vi "ArduinoMeasureWrite.vi"(0 "Arduino adress":refnum<visa-resource-name>="COM4", 4 "Measurement delay [s]":u32=5, 7 "error in":errorcluster) -> (17 "Average RH [%]":dbl, 19 "Average temperature [°C]":dbl, 21 "Temperature [°C]":dbl, 22 "Min temperature [°C]":dbl, 23 "Max temperature [°C]":dbl, 24 "Rel. Humidity [%]":dbl, 25 "Min RH [%]":dbl, 26 "Max RH [%]":dbl, 27 "error out":errorcluster)   [LabVIEW 2018]
doc: "Reads temperature and rel. humidity using arduino and creates a waveform graph with while loop iteration number on the x-axis, temperature on y1 axis and rel. humidity on the y2 axis."
panel:
  out "time":string
  out "output file refnum":refnum<file>
  in  "Select folder to save data":path=path "C:/Users/itkstriplabview3/Documents/TRH"
  in  "stop":bool
  out "Start time":timestamp
  out "Temp. & RH":cluster{dbl[], dbl[]}[](graph)
  out "Last 10 measurements":string[][](table)
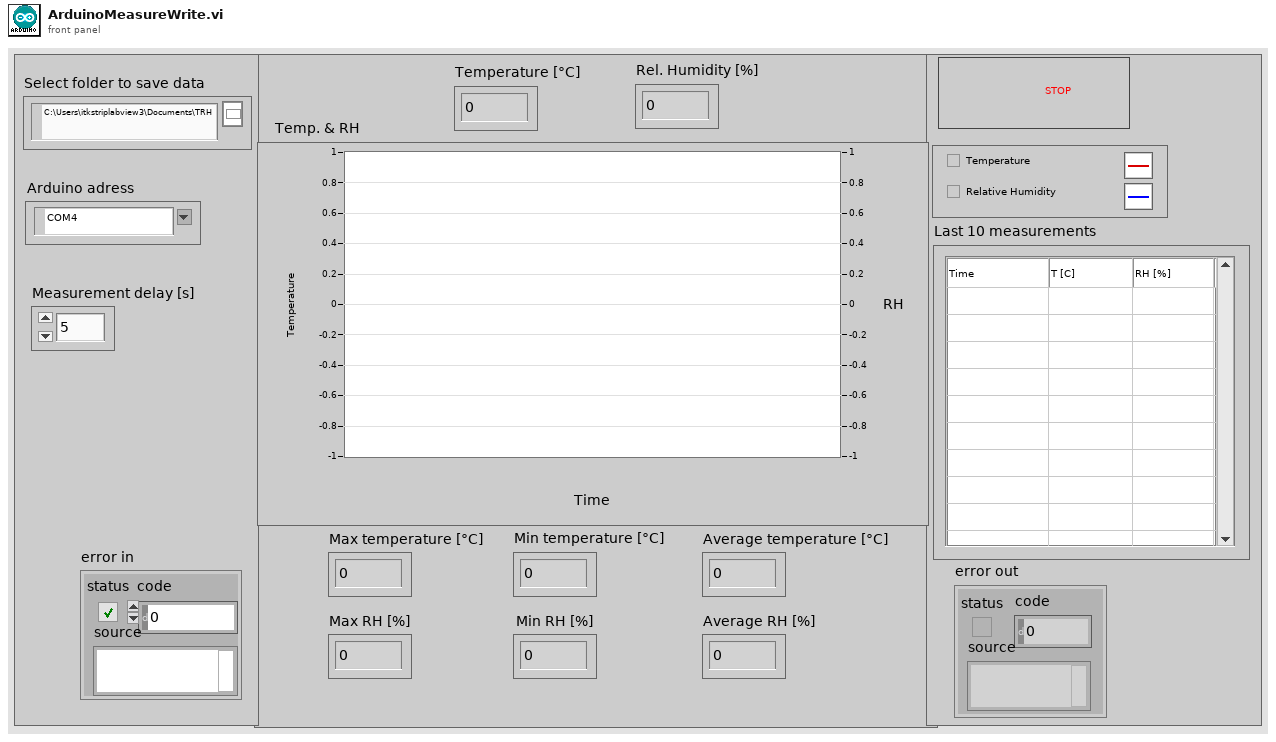
[diagram p1: front panel]
types:
  T1 = enum16{"open", "replace", "create", "open or create", "replace or create", "replace or create with confirmation"}
  T2 = typedef "LVDateTimeRec.ctl" = cluster{"fractional second":dbl, "second":i32, "minute":i32, "hour":i32, "day of month":i32, "month":i32, "year":i32, "day of week":i32, "day of year":i32, "DST":i32}
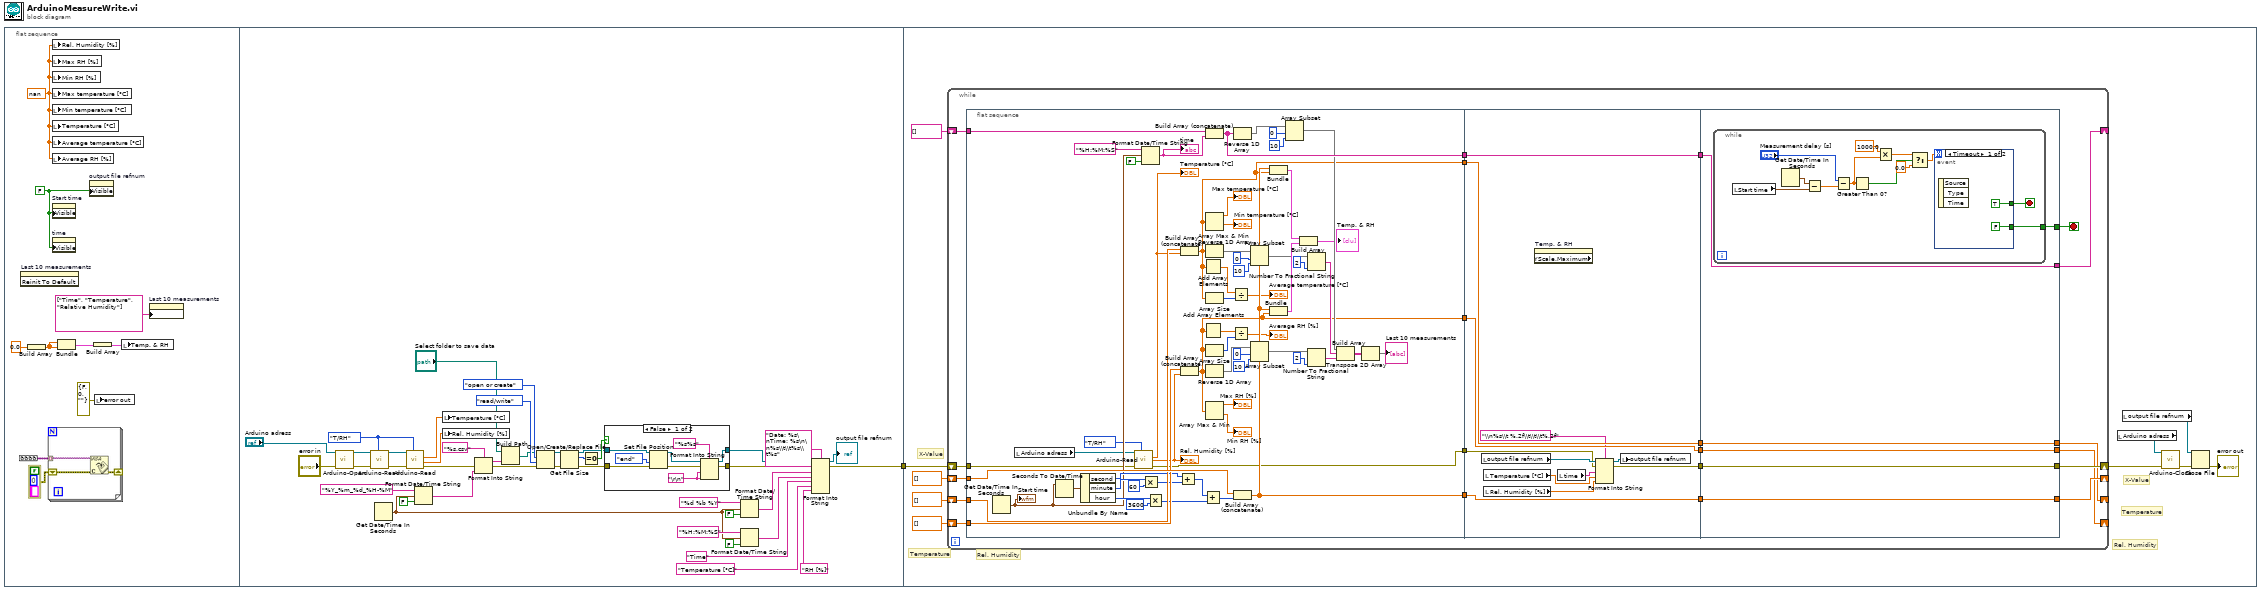
[diagram p0: block diagram]
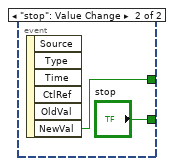
[diagram p3: hidden frame]
diagram:
  n1 = flat-sequence {
    tunnel: [w15] -> w1
    tunnel: w1 -> [w66]
    frame #0 {
      w3 = FALSE ("Visible")
      w6 = nan
      n2 = invoke on="Last 10 measurements" class="Tbl (strict)" method="Reinit To Default"() -> ()  [unwired: 3 in, 3 out]
      n3 = Build Array(0.0) -> (w8:dbl[])
      n4 = local write "Rel. Humidity [%]"(w6) -> ()
      n5 = local write "Max RH [%]"(w6) -> ()
      n6 = local write "Min RH [%]"(w6) -> ()
      n7 = local write "Max temperature [°C]"(w6) -> ()
      n8 = local write "Min temperature [°C]"(w6) -> ()
      n9 = local write "Temperature [°C]"(w6) -> ()
      n10 = local write "Average temperature [°C]"(w6) -> ()
      n11 = local write "Average RH [%]"(w6) -> ()
      n12 = property on="Start time" class="AbsTime (strict)"("Visible"=w3) -> ()  [unwired: 2 in, 2 out]
      n13 = property on="time" class="Str"("Visible"=w3) -> ()  [unwired: 2 in, 2 out]
      n14 = Bundle(w8, w8) -> (w7:cluster{dbl[], dbl[]})  [unwired: 1 in]
      n15 = property on="output file refnum" class="Ref (strict)"("Visible"=w3) -> ()  [unwired: 2 in, 2 out]
      n16 = Build Array(w7) -> (w9:cluster{dbl[], dbl[]}[])
      n17 = local write "error out"(errorcluster {"status"=FALSE, "code"=0, "source"=""} ("error out")) -> ()
      n18 = local write "Temp. & RH"(w9) -> ()
      n19 = property on="Last 10 measurements" class="Tbl (strict)"("Column Headers[]"=string[] ["Time", "Temperature", "Relative Humidity"]) -> ()  [unwired: 2 in, 2 out]
    }
    frame #1 {
      w42 = enum16{"T/RH", "Interlock", "Edgesense"}."T/RH" ("Arduino function")
      n20 = call "Arduino-Open.vi"("error in (no error)"="error in", "Visa Resource"="Arduino adress") -> ("error out"=w45:errorcluster, "VISA resource name out"=w47:refnum<visa-resource-name>)  [unwired: 7 in, 1 out]
      n21 = call "Arduino-Read.vi"("Arduino function"=w42, "error in (no error)"=w45, "VISA resource name"=w47) -> ("error out"=w46:errorcluster, "VISA resource name out"=w48:refnum<visa-resource-name>)  [unwired: 3 in, 4 out]
      n22 = Get Date/Time In Seconds() -> (seconds since 1Jan1904=w17:timestamp)
      n23 = call "Arduino-Read.vi"("Arduino function"=w42, "error in (no error)"=w46, "VISA resource name"=w48) -> ("error out"=w10:errorcluster, "rel. Humidity [%]"=w49:dbl, "Temperature [°C]"=w50:dbl)  [unwired: 3 in, 3 out]
      n24 = Format Date/Time String(time format string (%c)="%Y_%m_%d_%H-%M", seconds (now)=w17, UTC format=FALSE) -> (date/time string=w24:string)
      n25 = local write "Temperature [°C]"(w50) -> ()
      n26 = local write "Rel. Humidity [%]"(w49) -> ()
      n27 = Format Into String(format string="%s.csv", error in=w10, w24) -> (resulting string=w38:string, error out=w37:errorcluster)  [unwired: 1 in]
      n28 = Build Path(base path="Select folder to save data", name or relative path=w38) -> (appended path=w36:path)
      n29 = Open/Create/Replace File(file path (use dialog)=w36, error in=w37, operation (0:open)=T1."open or create", access (0:read/write)=enum16{"read/write", "read-only", "write-only"}."read/write") -> (refnum out=w34:refnum<file>, error out=w33:errorcluster)  [unwired: 2 in, 1 out]
      n30 = Get File Size(file=w34, error in=w33) -> (refnum out=w30:refnum<file>, size (in bytes)=w32:i64, 0:w29:errorcluster)
      n31 = Equal To 0?(x=w32) -> (x = 0?=w31:bool)
      n32 = case shown="False" w31 {
        tunnel: w30 -> [w59 w61]
        tunnel: w29 -> [w58 w60]
        tunnel: [w53 w61] -> w27
        tunnel: [w52 w60] -> w28
        frame False {
          w51 = "\r\n"
          n33 = Set File Position(refnum=w59, from (0:start)=enum16{"start", "end", "current"}."end", error in=w58) -> (refnum out=w55:refnum<file>, error out=w54:errorcluster)  [unwired: 1 in]
          n34 = Format Into String(format string="%s%s", initial string=w55, error in=w54, w51, w51) -> (resulting string=w53:refnum<file>, error out=w52:errorcluster)
        }
        frame True {
        }
      }
      n35 = Format Date/Time String(time format string (%c)="%d %b %Y", seconds (now)=w17, UTC format=FALSE) -> (date/time string=w21:string)
      n36 = Format Date/Time String(time format string (%c)="%H:%M:%S", seconds (now)=w17, UTC format=FALSE) -> (date/time string=w18:string)
      n37 = Format Into String(format string="Date: %s\nTime: %s\n\n%s\\t\\t%s\\t%s", initial string=w27, error in=w28, w21, w18, "Time" ("input 3"), "Temperature [°C]" ("input 4"), "RH [%]" ("input 5")) -> (resulting string=→"output file refnum":refnum<file>, error out=w15:errorcluster)
    }
    frame #2 {
      # "Rel. Humidity"
      # "Temperature"
      # "X-Value"
      # "Rel. Humidity"
      # "Temperature"
      # "X-Value"
      n38 = while {
        shift-right: [w92] -> w71
        shift-left: w66 -> [w88]
        shift-right: [w87] -> _
        shift-left: dbl[] [] -> [w91]
        shift-right: [w84] -> _
        shift-left: dbl[] [] -> [w90]
        shift-right: [w83] -> _
        shift-left: dbl[] [] -> [w89]
        shift-right: [w85] -> _
        shift-left: string[] [] -> [w86]
        stop <- w82 stop-if-true
        n39 = flat-sequence {
          tunnel: w91 -> [w151]
          tunnel: w90 -> [w150]
          tunnel: w89 -> [w149]
          tunnel: w88 -> [w97]
          tunnel: w86 -> [w119]
          tunnel: [w130] -> w80
          tunnel: [w115] -> w78
          tunnel: [w106] -> w76
          tunnel: [w102] -> w74
          tunnel: [w96] -> w72
          tunnel: [w155] -> w81
          tunnel: w80 -> [w163]
          tunnel: [w163] -> w79
          tunnel: w78 -> [w162]
          tunnel: [w162] -> w77
          tunnel: w76 -> [w161]
          tunnel: [w161] -> w75
          tunnel: w74 -> [w160]
          tunnel: [w160] -> w73
          tunnel: w72 -> [w152]
          tunnel: [w165] -> w83
          tunnel: [w166] -> w84
          tunnel: [w167] -> w85
          tunnel: [w168] -> w87
          tunnel: [w169] -> w92
          tunnel: w81 -> [w169]
          tunnel: w79 -> [w168]
          tunnel: w77 -> [w167]
          tunnel: w75 -> [w166]
          tunnel: w73 -> [w165]
          tunnel: [w164] -> w82
          frame #0 {
            n40 = Get Date/Time In Seconds() -> (seconds since 1Jan1904=w99:timestamp)
            "Start time" <- w99
            n41 = local read "Arduino adress"() -> (w93:refnum<visa-resource-name>)
            n42 = Seconds To Date/Time(time stamp (now)=w99) -> (date time rec=w140:T2)  [unwired: 1 in]
            n43 = Unbundle By Name(w140) -> ("second"=w137:i32, "minute"=w138:i32, "hour"=w134:i32)
            n44 = call "Arduino-Read.vi"("Arduino function"=enum16{"T/RH", "Interlock", "Edgesense"}."T/RH", "error in (no error)"=w97, "VISA resource name"=w93) -> ("error out"=w96:errorcluster, "rel. Humidity [%]"=w146:dbl, "Temperature [°C]"=w145:dbl)  [unwired: 3 in, 3 out]
            "Rel. Humidity [%]" <- w146
            "Temperature [°C]" <- w145
            n45 = Format Date/Time String(time format string (%c)="%H:%M:%S", seconds (now)=w99, UTC format=FALSE) -> (date/time string=w98:string)
            "time" <- w98
            n46 = Multiply(x=w138, y=60) -> (x*y=w136:i32)
            n47 = Multiply(x=w134, y=3600) -> (x*y=w133:i32)
            n48 = Add(x=w137, y=w136) -> (x+y=w132:i32)
            n49 = Build Array (concatenate)(w150, w145) -> (w106:dbl[])
            n50 = Build Array (concatenate)(w149, w146) -> (w102:dbl[])
            n51 = Add Array Elements(numeric array=w106) -> (sum=w107:dbl)
            n52 = Add Array Elements(numeric array=w102) -> (sum=w103:dbl)
            n53 = Add(x=w132, y=w133) -> (x+y=w131:i32)
            n54 = Build Array (concatenate)(w119, w98) -> (w115:string[])
            n55 = Array Max & Min(array=w106) -> (max value=→"Max temperature [°C]":dbl, min value=→"Min temperature [°C]":dbl)  [unwired: 2 out]
            n56 = Reverse 1D Array(array=w106) -> (reversed array=w127:dbl[])
            n57 = Array Size(array=w106) -> (size(s)=w108:i32)
            n58 = Array Size(array=w102) -> (size(s)=w104:i32)
            n59 = Reverse 1D Array(array=w102) -> (reversed array=w124:dbl[])
            n60 = Array Max & Min(array=w102) -> (max value=→"Max RH [%]":dbl, min value=→"Min RH [%]":dbl)  [unwired: 2 out]
            n61 = Divide(x=w107, y=w108) -> (x/y=→"Average temperature [°C]":dbl)
            n62 = Divide(x=w103, y=w104) -> (x/y=→"Average RH [%]":dbl)
            n63 = Reverse 1D Array(array=w115) -> (reversed array=w116:string[])
            n64 = Build Array (concatenate)(w151, w131) -> (w130:dbl[])
            n65 = Array Subset(array=w127, index=0, length=10) -> (w121:dbl[])
            n66 = Array Subset(array=w124, index=0, length=10) -> (w123:dbl[])
            n67 = Bundle(w130, w106) -> (w148:cluster{dbl[], dbl[]})  [unwired: 1 in]
            n68 = Bundle(w130, w102) -> (w147:cluster{dbl[], dbl[]})  [unwired: 1 in]
            n69 = Array Subset(array=w116, index=0, length=10) -> (w114:string[])
            n70 = Build Array(w148, w147) -> (→"Temp. & RH":cluster{dbl[], dbl[]}[])
            n71 = Number To Fractional String(number=w121, precision (6)=i16 2) -> (F-format string=w113:string[])  [unwired: 2 in]
            n72 = Number To Fractional String(number=w123, precision (6)=i16 2) -> (F-format string=w112:string[])  [unwired: 2 in]
            n73 = Build Array(w114, w113, w112) -> (w111:string[][])
            n74 = Transpose 2D Array(2D array=w111) -> (transposed array=→"Last 10 measurements":string[][])
          }
          frame #1 {
            n75 = local read "output file refnum"() -> (w153:refnum<file>)
            n76 = local read "Temperature [°C]"() -> (w157:dbl)
            n77 = local read "Rel. Humidity [%]"() -> (w156:dbl)
            n78 = property on="Temp. & RH" class="XYGraph (strict)" props=["YScale", "Maximum"]() -> ()  [unwired: 2 in, 3 out]
            n79 = local read "time"() -> (w158:string)
            n80 = Format Into String(format string="\\n%s\\t %.2f\\t\\t\\t%.2f", initial string=w153, error in=w152, w158, w157, w156) -> (resulting string=w154:refnum<file>, error out=w155:errorcluster)
            n81 = local write "output file refnum"(w154) -> ()
          }
          frame #2 {
            n82 = while {
              tunnel: [w170] -> w164
              stop <- w171 stop-if-true
              n83 = local read "Start time"() -> (w180:timestamp)
              n84 = Get Date/Time In Seconds() -> (seconds since 1Jan1904=w181:timestamp)
              n85 = Subtract(x=w181, y=w180) -> (x-y=w178:dbl)
              n86 = Subtract(x="Measurement delay [s]", y=w178) -> (x-y=w175:dbl)
              n87 = Greater Than 0?(x=w175) -> (x > 0?=w177:bool)
              n88 = Multiply(x=1000.0, y=w175) -> (x*y=w173:dbl)
              n89 = Select(t=w173, s=w177, f=0.0) -> (s? t:f=w172:dbl)
              n90 = event shown="[0] Timeout" {
                selector: _ -> [_ _]
                dyn-events: _ -> [_ _]
                timeout: w172 -> [_ _]
                tunnel: [TRUE w185] -> w171
                tunnel: [FALSE "stop"] -> w170
                event Timeout {
                  n91 = event-data() -> ()  [unwired: 1 in, 3 out]
                }
                event "stop": Value Change {
                  n92 = event-data() -> ("NewVal"=w185:bool)  [unwired: 1 in, 5 out]
                }
              }
            }
          }
        }
      }
      n93 = local read "Arduino adress"() -> (w65:refnum<visa-resource-name>)
      n94 = local read "output file refnum"() -> (w62:refnum<file>)
      n95 = call "Arduino-Close.vi"("error in (no error)"=w71, "VISA resource name"=w65) -> ("error out"=w64:errorcluster)  [unwired: 9 in]
      n96 = Close File(refnum=w62, error in=w64) -> (error out=→"error out":errorcluster)  [unwired: 1 out]
    }
  }
